vi "Read.vi"(8 "error in (no error)":errorcluster, 9 "Timeout":u32, 10 "Last message":refnum<class "BaseMessage.lvclass">, 11 "MultiReader in":refnum<class "MultiReader.lvclass">) -> (0 "error out":errorcluster, 1 "isAck?":bool, 2 "Responses":T1[](array[typedef]), 3 "MultiReader out":refnum<class "MultiReader.lvclass">)   [LabVIEW 2013, in "MultiReader.lvclass"]
doc: "Read a message from the remote destination"
uses:
  MultiReader.lvclass
  Message/BaseMessage/BaseMessage.lvclass
  response.ctl
  driver_status.ctl
  MultiReader.lvclass/MultiReader.ctl
  BaseReader/BaseReader.lvclass
  BaseReader/BaseReader.lvclass/BaseReader.ctl
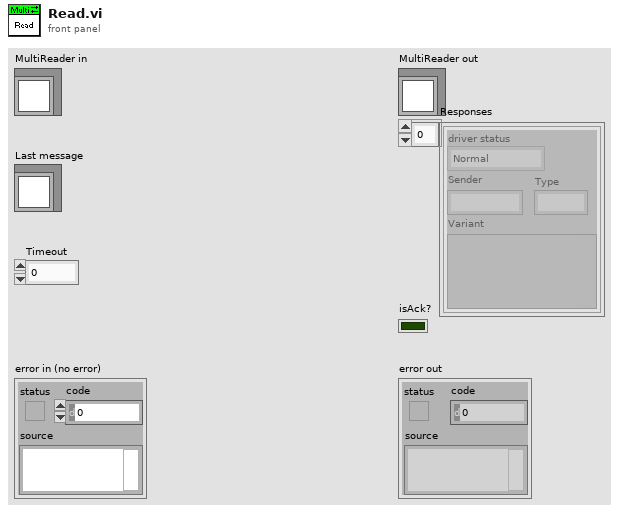
[diagram p1: front panel]
types:
  T1 = typedef "response.ctl" = cluster{"driver status":T2, "Sender":string, "Type":i32, "Variant":variant}
  T2 = typedef "driver_status.ctl" = enum16{"Normal", "Startup", "Connection lost", "Reconnected", "Timeout", "Idle", "Busy"}
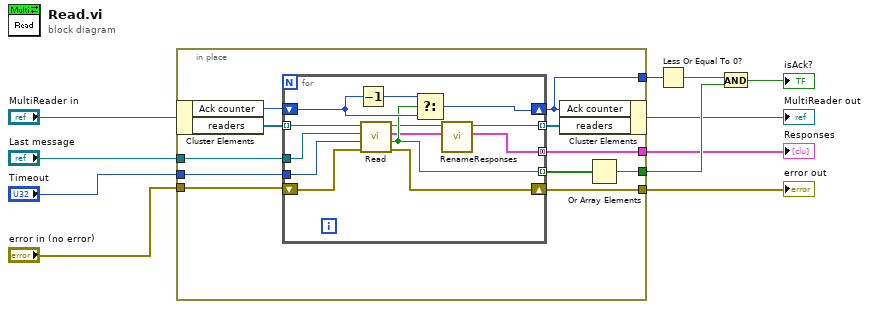
[diagram p0: block diagram]
diagram:
  n1 = in-place {
    in-place-border: "error in (no error)" -> [w20]
    in-place-border: [w19] -> w1
    in-place-border: "Last message" -> [w18]
    in-place-border: [w17] -> w2
    in-place-border: "Timeout" -> [w16]
    in-place-border: [w14] -> w7
    in-place-border: [w12] -> w5
    n2 = in-place-cluster #1("MultiReader in") -> ("Ack counter"=w15:i32, "readers"=w22:refnum<class "BaseReader.lvclass">[])
    n3 = for {
      tunnel: w22 -> [w35] mode=indexing
      tunnel: [w24] -> w21 mode=indexing
      shift-right: [w32] -> w19
      shift-left: w20 -> [w33]
      tunnel: w18 -> [w34]
      tunnel: [w23] -> w17 mode=concatenating
      tunnel: w16 -> [w31]
      shift-right: [w29] -> w14
      shift-left: w15 -> [w28]
      tunnel: [w27] -> w13 mode=indexing
      n4 = Decrement(x=w28) -> (x-1=w30:i32)
      n5 = call-dynamic "Read.vi"("error in (no error)"=w33, "Timeout"=w31, "Last message"=w34, "BaseReader in"=w35) -> ("error out"=w32:errorcluster, "isAck?"=w27:bool, "Responses"=w25:T1[], "BaseReader out"=w26:refnum<class "BaseReader.lvclass">)  [unwired: 4 in]
      n6 = Select(t=w30, s=w27, f=w28) -> (s? t:f=w29:i32)
      n7 = call "RenameResponses.vi"("Responses"=w25, "BaseReader in"=w26) -> ("Responses out"=w23:T1[], "BaseReader out"=w24:refnum<class "BaseReader.lvclass">)  [unwired: 7 in, 1 out]
    }
    n8 = in-place-cluster #1("Ack counter"=w14, "readers"=w21) -> (→"MultiReader out":refnum<class "MultiReader.lvclass">)
    n9 = Or Array Elements(Boolean array=w13) -> (logical OR=w12:bool)
  }
  "error out" <- w1
  "Responses" <- w2
  n10 = Less Or Equal To 0?(x=w7) -> (x <= 0?=w6:bool)
  n11 = And(x=w6, y=w5) -> (x .and. y?=→"isAck?":bool)
